vi "Get Histogram Low & High Percentile Locations.vi"(8 "Error In":errorcluster, 9 "Lower Percentile [0-100], Default: 5":dbl=5.0 min=0.0 max=100.0, 10 "Upper Percentile [0-100], Default: 95":dbl=95.0 min=0.0 max=100.0, 11 "Histogram":cluster{"Axis":dbl[], "Histogram":dbl[]}) -> (0 "Error Out":errorcluster, 1 "Lower Percentile Location":dbl, 3 "Upper Percentile Location":dbl, 4 "Lower Percentile Bin":dbl, 5 "Upper Percentile Bin":dbl)   [LabVIEW 2021, in "Histograms.lvlib"]
uses:
  Histograms.lvlib
  3a60366f-bb0f-4610-9615-1ec8c8b0bc54.vi
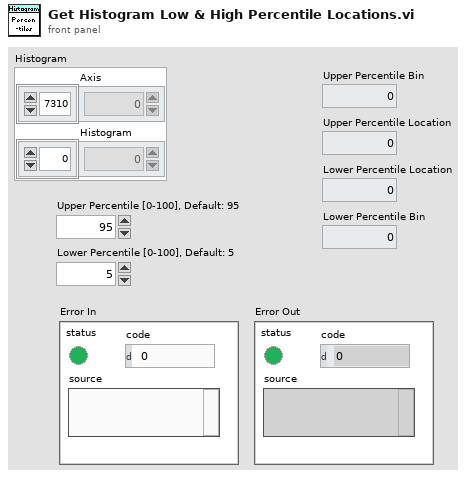
[diagram p1: front panel]
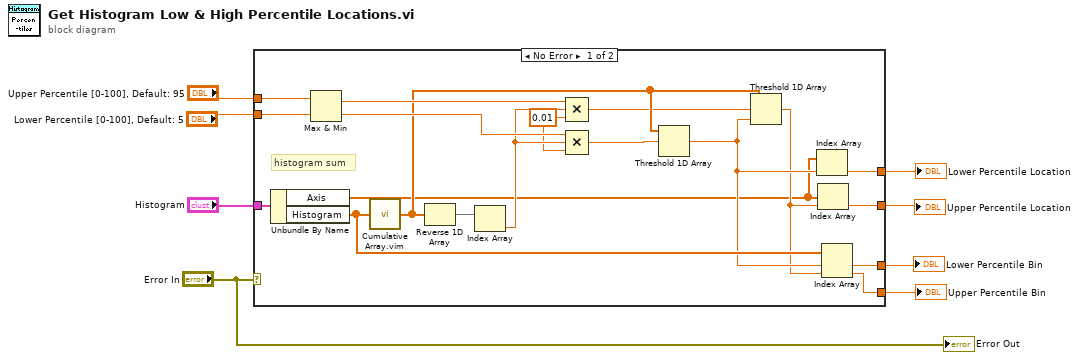
[diagram p0: block diagram]
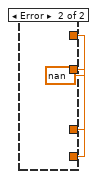
[diagram p2: hidden frame]
diagram:
  n1 = case shown="No Error" "Error In" {
    tunnel: "Histogram" -> [w27 _]
    tunnel: "Upper Percentile [0-100], Default: 95" -> [w25 _]
    tunnel: "Lower Percentile [0-100], Default: 5" -> [w24 _]
    tunnel: [w12 w28] -> w6
    tunnel: [w10 w28] -> w5
    tunnel: [w15 w28] -> w3
    tunnel: [w14 w28] -> w2
    frame No Error {
      w20 = 0.01 ("value")
      # "histogram sum"
      n2 = Unbundle By Name(w27) -> ("Axis"=w9:dbl[], "Histogram"=w16:dbl[])
      n3 = Max & Min(x=w25, y=w24) -> (max(x,y)=w23:dbl, min(x,y)=w22:dbl)
      n4 = call "Cumulative Array.vim"("Array"=w16) -> ("cumulative Array"=w18:dbl[])  [unwired: 8 in]
      n5 = Reverse 1D Array(array=w18) -> (reversed array=w26:dbl[])
      n6 = Index Array(array=w26) -> (element=w21:dbl)  [unwired: 1 in]
      n7 = Compound Arithmetic op=MULTIPLY(w23, w21, w20) -> (w17:dbl)
      n8 = Compound Arithmetic op=MULTIPLY(w22, w21, w20) -> (w19:dbl)
      n9 = Threshold 1D Array(2:w19, 3:w18) -> (0:w13:dbl)  [unwired: 1 in]
      n10 = Threshold 1D Array(1:w13, 2:w17, 3:w18) -> (0:w11:dbl)
      n11 = Index Array(array=w9, index=w13) -> (element=w12:dbl)
      n12 = Index Array(array=w9, index=w11) -> (element=w10:dbl)
      n13 = Index Array(array=w16, index #1=w13, index #2=w11) -> (element #1=w15:dbl, element #2=w14:dbl)
    }
    frame Error {
      w28 = nan ("Numeric")
    }
  }
  "Lower Percentile Location" <- w6
  "Upper Percentile Location" <- w5
  "Lower Percentile Bin" <- w3
  "Upper Percentile Bin" <- w2
  "Error Out" <- "Error In"
